vi "New BrowerTree.vi"(8 "error in (no error)":errorcluster, 10 "Tree Refnum":refnum<vi>, 11 "BrowerTree in":refnum<class "BrowerTree.lvclass">) -> (0 "error out":errorcluster, 3 "BrowerTree out":refnum<class "BrowerTree.lvclass">)   [LabVIEW 2015, in "BrowerTree.lvclass"]
uses:
  BrowerTree.lvclass
  BrowerTree.lvclass/BrowerTree.ctl
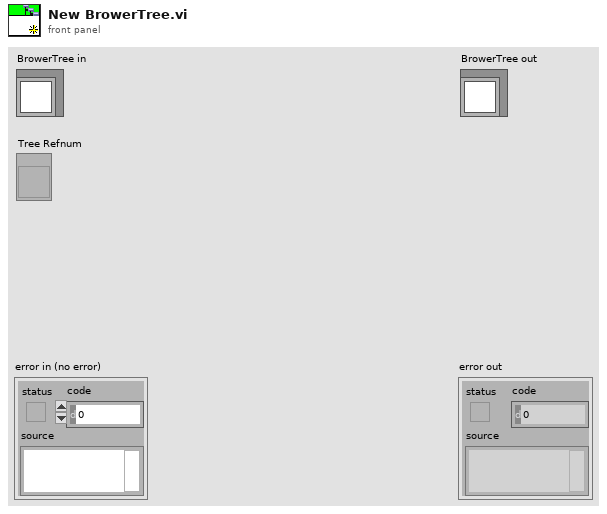
[diagram p1: front panel]
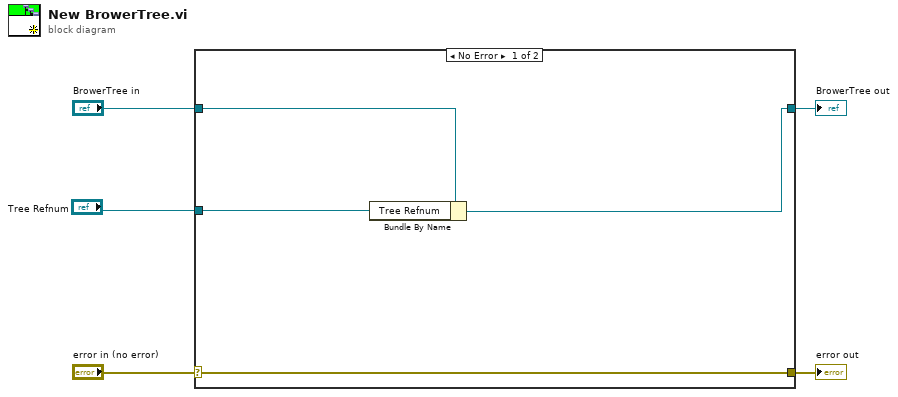
[diagram p0: block diagram]
diagram:
  n1 = case shown="No Error" "error in (no error)" {
    selector: "error in (no error)" -> [w9 w11]
    tunnel: [w9 w11] -> w4
    tunnel: [w7 w10] -> w2
    tunnel: "BrowerTree in" -> [w8 w10]
    tunnel: "Tree Refnum" -> [w6 _]
    frame No Error {
      n2 = Bundle By Name(cluster=w8, "Tree Refnum"=w6) -> (w7:refnum<class "BrowerTree.lvclass">)
    }
    frame Error {
    }
  }
  "error out" <- w4
  "BrowerTree out" <- w2
